vi "ORS_GalvoInit2_uw.vi"(4 "acq trig out an":tag="Dev1/ao2" caption="Acq trig out an", 5 "acq trig out":tag="Dev1/port0/line4" caption="Acq trig out", 6 "custom trig out":tag="Dev1/port0/line7" caption="Custom trigger out", 7 "Galvo Clk input":tag="/Dev1/PFI0", 8 "error in":errorcluster, 9 "trig out":tag="Dev1/port0/line2" caption="Trigger AND output", 10 "y mirror":tag="Dev1/ao1" caption="Y mirror analog out", 11 "x mirror":tag="Dev1/ao0" caption="X mirror analog out") -> (0 "error out":errorcluster, 3 "Galvo out":T1={"x mirror"="Dev1/ao0", "y mirror"="Dev1/ao1", "trig out"="Dev1/port0/line2", "x mirror task"="", "y mirror task"="", "trig out task"="", "n_axis"=0, "params"={"n_lines"=0, "n_frames"=0, "force to zero"=FALSE, "Triggers_per_sweep"=0.0, "X center"=0.0, "X span"=0.0, "Y center"=0.0, "Y span"=0.0, "flyb.lines"=0, "n_triggers"=0, "mode"=0, "offset"=0.0, "galvo phase"=0, "span factor"=0.0, "Custom trig."={"n_f to c. trig"=0, "c. trig length"=0, "c. trig interval"=0, "n_c. trig"=0}, "f_per_pos"=0, "n_dataset"=0, "flyback fr"=0}, "acq trig out"="Dev1/port0/line4", "acq trig out task"="", "sample array X"=[], "sample array Y"=[], "custom trig out"="", "custom trig out task"="", "FDML-box"="TCPIP0::10.153.218.51::23::SOCKET", "ACQ/Galvo"=enum."ADC/FDML", "acq trig out an task"="", "acq trig out an"="Dev1/ao2", "Galvo Trig input"="/Dev1/PFI0", "Galvo Clk input"="/Dev1/PFI0", "sample array Acq trig out an"=[]} {"params"."n_dataset" min=1; "params"."X center" format="%^_3g"; "params"."X span" format="%^_3g"; "params"."Y center" format="%^_3g"; "params"."Y span" format="%^_3g"})   [LabVIEW 2024]
uses:
  typedef/ORS_Galvo.ctl
  typedef/ORS_Galvo_params.ctl
  <vilib>/DAQmx/write.llb/DAQmx Write (Digital 1D Bool NChan 1Samp 1Line).vi
  <vilib>/DAQmx/write.llb/DAQmx Write (Digital Bool 1Line 1Point).vi
  <vilib>/DAQmx/create/channels.llb/DAQmx Create Channel (DO-Digital Output).vi
  <vilib>/DAQmx/miscellaneous.llb/DAQmx Fill In Error Info.vi
panel:
  in  "Galvo Trigger input":tag="/Dev1/PFI1" caption="Galvo Trig input"
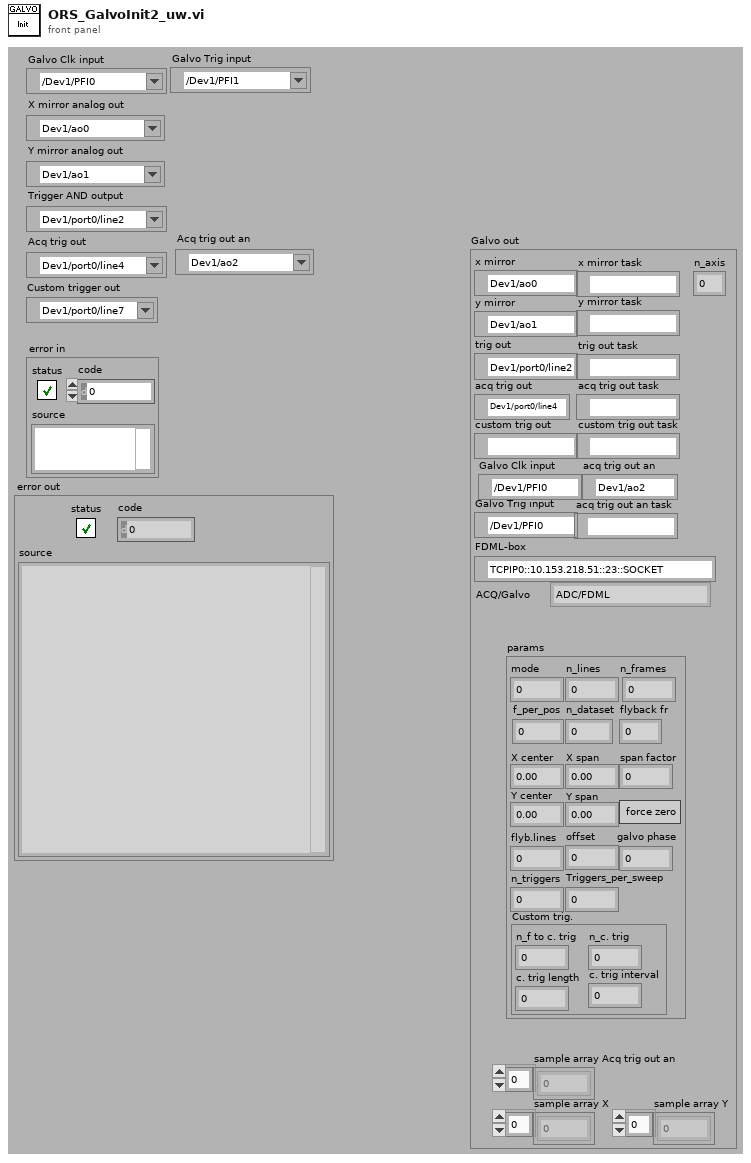
[diagram p1: front panel]
types:
  T1 = typedef "ORS_Galvo.ctl" = cluster{"x mirror":tag, "y mirror":tag, "trig out":tag, "x mirror task":refnum<k21>, "y mirror task":refnum<k21>, "trig out task":refnum<k21>, "n_axis":i32, "params":T2, "acq trig out":tag, "acq trig out task":refnum<k21>, "sample array X":dbl[], "sample array Y":dbl[], "custom trig out":tag, "custom trig out task":refnum<k21>, "FDML-box":refnum<visa-resource-name>, "ACQ/Galvo":enum16{"ADC/FDML", "NI_DAQ", "ADC"}, "acq trig out an task":refnum<k21>, "acq trig out an":tag, "Galvo Trig input":tag, "Galvo Clk input":tag, "sample array Acq trig out an":dbl[]}
  T2 = typedef "ORS_Galvo_params.ctl" = cluster{"n_lines":i32, "n_frames":i32, "force to zero":bool, "Triggers_per_sweep":dbl, "X center":dbl, "X span":dbl, "Y center":dbl, "Y span":dbl, "flyb.lines":i32, "n_triggers":i32, "mode":i32, "offset":dbl, "galvo phase":i32, "span factor":dbl, "Custom trig.":cluster{"n_f to c. trig":i32, "c. trig length":i32, "c. trig interval":i32, "n_c. trig":i32}, "f_per_pos":i32, "n_dataset":u32, "flyback fr":u16}
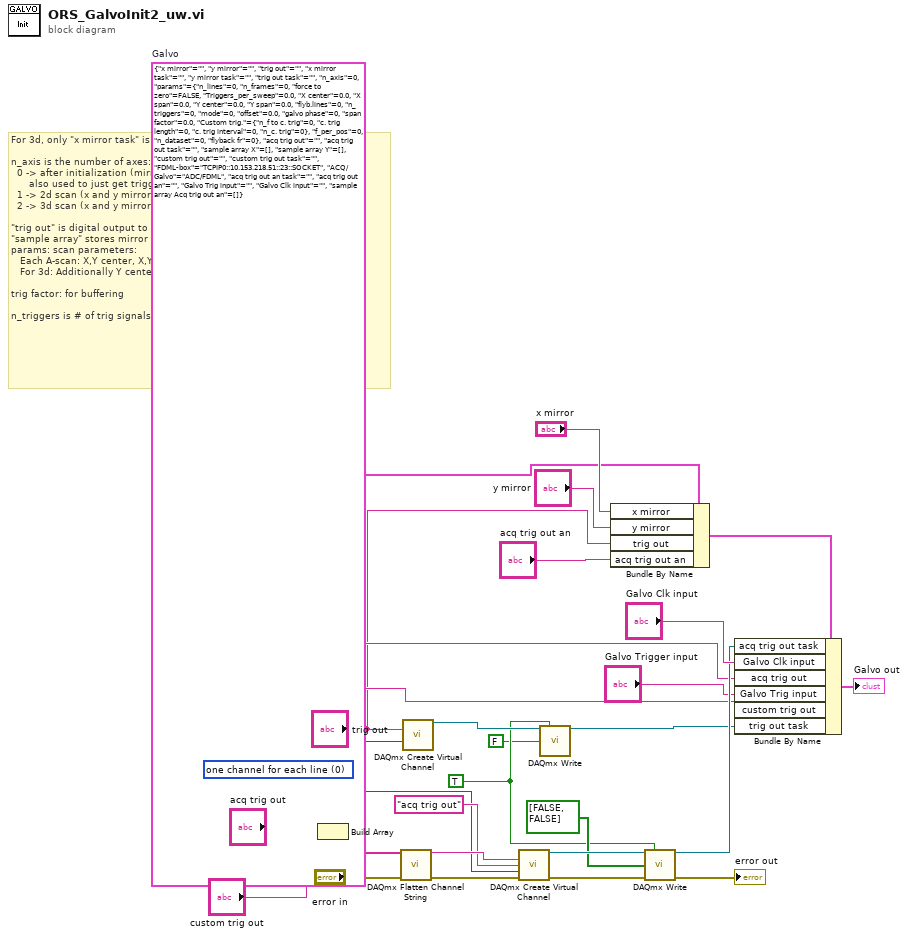
[diagram p0: block diagram]
diagram:
  w14 = T1 {"x mirror"="", "y mirror"="", "trig out"="", "x mirror task"="", "y mirror task"="", "trig out task"="", "n_axis"=0, "params"={"n_lines"=0, "n_frames"=0, "force to zero"=FALSE, "Triggers_per_sweep"=0.0, "X center"=0.0, "X span"=0.0, "Y center"=0.0, "Y span"=0.0, "flyb.lines"=0, "n_triggers"=0, "mode"=0, "offset"=0.0, "galvo phase"=0, "span factor"=0.0, "Custom trig."={"n_f to c. trig"=0, "c. trig length"=0, "c. trig interval"=0, "n_c. trig"=0}, "f_per_pos"=0, "n_dataset"=0, "flyback fr"=0}, "acq trig out"="", "acq trig out task"="", "sample array X"=[], "sample array Y"=[], "custom trig out"="", "custom trig out task"="", "FDML-box"="TCPIP0::10.153.218.51::23::SOCKET", "ACQ/Galvo"=enum."ADC/FDML", "acq trig out an task"="", "acq trig out an"="", "Galvo Trig input"="", "Galvo Clk input"="", "sample array Acq trig out an"=[]}  # Galvo
  w5 = 0 items=["one channel for each line", "one channel for all lines"] ("line grouping")
  w3 = TRUE ("auto start")
  # "For 3d, only \"x mirror task\" is used as task for both mirrors. \n\nn_axis is the number of axes: \n  0 -> after initialization (mirror tasks are invalid)\n      also used to just get triggers for background acq and similar.\n  1 -> 2d scan (x and y mirror task active)\n  2 -> 3d scan (x and y mirror correlated both using \"x mirror task\")\n\n\"trig out\" is digital output to trigger mirrors and acquisition card.\n\"sample array\" stores mirror samples for 2d (n_axis=1) only. \nparams: scan parameters:\n   Each A-scan: X,Y center, X,Y span; for 2d: n_lines (Y pos no loger used)\n   For 3d: Additionally Y center, Y span, n_frames\n\ntrig factor: for buffering\n\nn_triggers is # of trig signals to generate for n_axis=0 scan."
  n1 = Build Array("acq trig out", "custom trig out") -> (w18:tag[])
  n2 = call <vilib>:"DAQmx Flatten Channel String.vi"("names in"=w18, "error in"="error in") -> ("names out"=w17:string, "error out"=w20:errorcluster)  [unwired: 12 in]
  n3 = call-poly <vilib>:"DAQmx Create Virtual Channel.vi"("lines"="trig out", "line grouping"=w5) -> ("task out"=w4:refnum<k21>)  [unwired: 12 in, 1 out]
  n4 = call-poly <vilib>:"DAQmx Create Virtual Channel.vi"("lines"=w17, "name to assign"="acq trig out", "line grouping"=w5, "error in"=w20) -> ("task out"=w23:refnum<k21>, "error out"=w22:errorcluster)  [unwired: 10 in]
  n5 = call-poly <vilib>:"DAQmx Write.vi"("task/channels in"=w4, "auto start"=w3, "data"=FALSE) -> ("task out"=w1:refnum<k21>)  [unwired: 10 in, 2 out]
  n6 = Bundle By Name(cluster=w14, "x mirror"="x mirror", "y mirror"="y mirror", "trig out"="trig out", "acq trig out an"="acq trig out an") -> (w24:T1)
  n7 = call-poly <vilib>:"DAQmx Write.vi"("task/channels in"=w23, "auto start"=w3, "data"=bool[] [FALSE, FALSE], "error in"=w22) -> ("task out"=w16:refnum<k21>, "error out"=→"error out":errorcluster)  [unwired: 9 in, 1 out]
  n8 = Bundle By Name(cluster=w24, "acq trig out task"=w16, "Galvo Clk input"="Galvo Clk input", "acq trig out"="acq trig out", "Galvo Trig input"="Galvo Trigger input", "custom trig out"="custom trig out", "trig out task"=w1) -> (→"Galvo out":T1)
